vi "Read Libraries.vi"(11 "ProjectItem in":refnum<class "ProjectItem.lvclass">) -> (2 "Libraries":T1, 3 "ProjectItem out":refnum<class "ProjectItem.lvclass">)   [LabVIEW 2016, in "ProjectItem.lvclass"]
uses:
  ProjectItem.lvclass
  ProjectItem.lvclass/ProjectItem.ctl
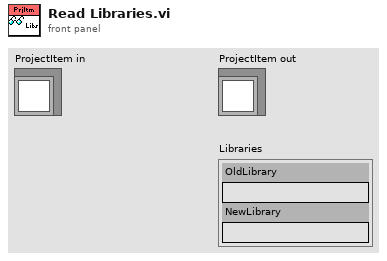
[diagram p1: front panel]
types:
  T1 = cluster{"OldLibrary":string, "NewLibrary":string}
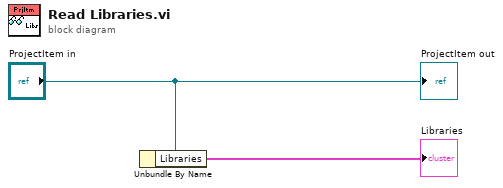
[diagram p0: block diagram]
diagram:
  n1 = Unbundle By Name("ProjectItem in") -> ("Libraries"=→"Libraries":T1)
  "ProjectItem out" <- "ProjectItem in"
